vi "PLC.CheckStatus.vi"(7 "Idx":i32, 8 "error in":errorcluster, 10 "Slot":i32, 11 "Data_in":T1={"Status"={"Idx"=0, "ConnRef"=0, "State"=enum."Off", "LiveBitTimer"=timestamp(0 s since 1904-01-01)}, "Sets"={"Enable"=FALSE, "IP"="", "Rack"=0, "Slot"=0, "LifeBitTimer_s"=0.0, "DataBlockAddr_PCStatus"=0, "DataBlockAddr_PLCStatus"=1, "DataBlockAddr_PLCNewData"=[], "DataBlockSize_PLCNewData"=[], "DataBlockAddr_PLCChangeOver"=[], "DataBlockSize_PLCChangeOver"=[], "DataBlockAddr_PCChangeOver"=[], "DataBlockAddr_PLCCheckStatus"=[], "DataBlockSize_PLCCheckStatus"=[], "DataBlockAddr_PCCheckStatus"=[], "System"=""}, "PCstatus"={"General"={"LifeBit"=FALSE, "DbRun"=FALSE}, "Stations"=[]}, "PLCstatus"={"General"={"LifeBit"=FALSE}, "Stations"=[]}}) -> (0 "error out":errorcluster, 3 "Data_out":T1={"Status"={"Idx"=0, "ConnRef"=0, "State"=enum."Off", "LiveBitTimer"=timestamp(0 s since 1904-01-01)}, "Sets"={"Enable"=FALSE, "IP"="", "Rack"=0, "Slot"=0, "LifeBitTimer_s"=0.0, "DataBlockAddr_PCStatus"=0, "DataBlockAddr_PLCStatus"=1, "DataBlockAddr_PLCNewData"=[], "DataBlockSize_PLCNewData"=[], "DataBlockAddr_PLCChangeOver"=[], "DataBlockSize_PLCChangeOver"=[], "DataBlockAddr_PCChangeOver"=[], "DataBlockAddr_PLCCheckStatus"=[], "DataBlockSize_PLCCheckStatus"=[], "DataBlockAddr_PCCheckStatus"=[], "System"=""}, "PCstatus"={"General"={"LifeBit"=FALSE, "DbRun"=FALSE}, "Stations"=[]}, "PLCstatus"={"General"={"LifeBit"=FALSE}, "Stations"=[]}})   [LabVIEW 2016]
doc: "Get test results (measurement values) from PLC and save to database\n\nWabco 2017 All right reserved\nAuthor: maciej.szupienko@wabco-auto.com"
uses:
  PLC.Data.ctl
  PLC.Data.Status.ctl
  PLC.State.ctl
  PLC.Data.Sets.ctl
  LowLevel/PLC.DataBlock.PCstatus.ctl
  LowLevel/PLC.DataBlock.PCstatus.General.ctl
  LowLevel/PLC.DataBlock.PCstatus.Station.ctl
  LowLevel/PLC.DataBlock.PLCstatus.ctl
  LowLevel/PLC.DataBlock.PLCstatus.General.ctl
  LowLevel/PLC.DataBlock.PLCstatus.Station.ctl
  LowLevel/PLC.DataBlock.PLCcheckstatus.ctl
  LowLevel/PLC.DataBlock.PCcheckstatus.ctl
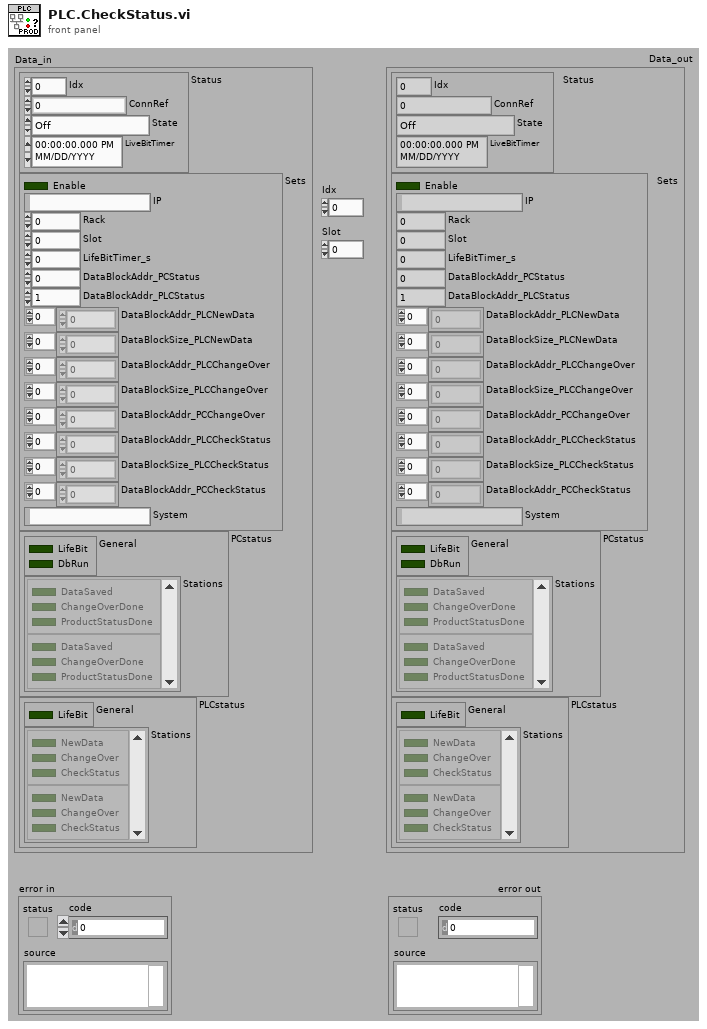
[diagram p1: front panel]
types:
  T1 = typedef "PLC.Data.ctl" = cluster{"Status":T2, "Sets":T4, "PCstatus":T5, "PLCstatus":T8}
  T2 = typedef "PLC.Data.Status.ctl" = cluster{"Idx":i32, "ConnRef":u64, "State":T3, "LiveBitTimer":timestamp}
  T3 = typedef "PLC.State.ctl" = enum32{"Off", "Error", "Idle", "Run"}
  T4 = typedef "PLC.Data.Sets.ctl" = cluster{"Enable":bool, "IP":string, "Rack":i32, "Slot":i32, "LifeBitTimer_s":dbl, "DataBlockAddr_PCStatus":i32, "DataBlockAddr_PLCStatus":i32, "DataBlockAddr_PLCNewData":i32[], "DataBlockSize_PLCNewData":i32[], "DataBlockAddr_PLCChangeOver":i32[], "DataBlockSize_PLCChangeOver":i32[], "DataBlockAddr_PCChangeOver":i32[], "DataBlockAddr_PLCCheckStatus":i32[], "DataBlockSize_PLCCheckStatus":i32[], "DataBlockAddr_PCCheckStatus":i32[], "System":string}
  T5 = typedef "PLC.DataBlock.PCstatus.ctl" = cluster{"General":T6, "Stations":T7[]}
  T6 = typedef "PLC.DataBlock.PCstatus.General.ctl" = cluster{"LifeBit":bool, "DbRun":bool}
  T7 = typedef "PLC.DataBlock.PCstatus.Station.ctl" = cluster{"DataSaved":bool, "ChangeOverDone":bool, "ProductStatusDone":bool}
  T8 = typedef "PLC.DataBlock.PLCstatus.ctl" = cluster{"General":T9, "Stations":T10[]}
  T9 = typedef "PLC.DataBlock.PLCstatus.General.ctl" = cluster{"LifeBit":bool}
  T10 = typedef "PLC.DataBlock.PLCstatus.Station.ctl" = cluster{"NewData":bool, "ChangeOver":bool, "CheckStatus":bool}
  T11 = typedef "PLC.DataBlock.PCcheckstatus.ctl" = cluster{"Ref":string, "Serial":string, "StatusPrev":i8, "StatusThis":i8, "Repetitions":u8}
  T12 = typedef "PLC.DataBlock.PLCcheckstatus.ctl" = cluster{"Ref1":string, "Serial1":string, "Ref2":string, "Serial2":string}
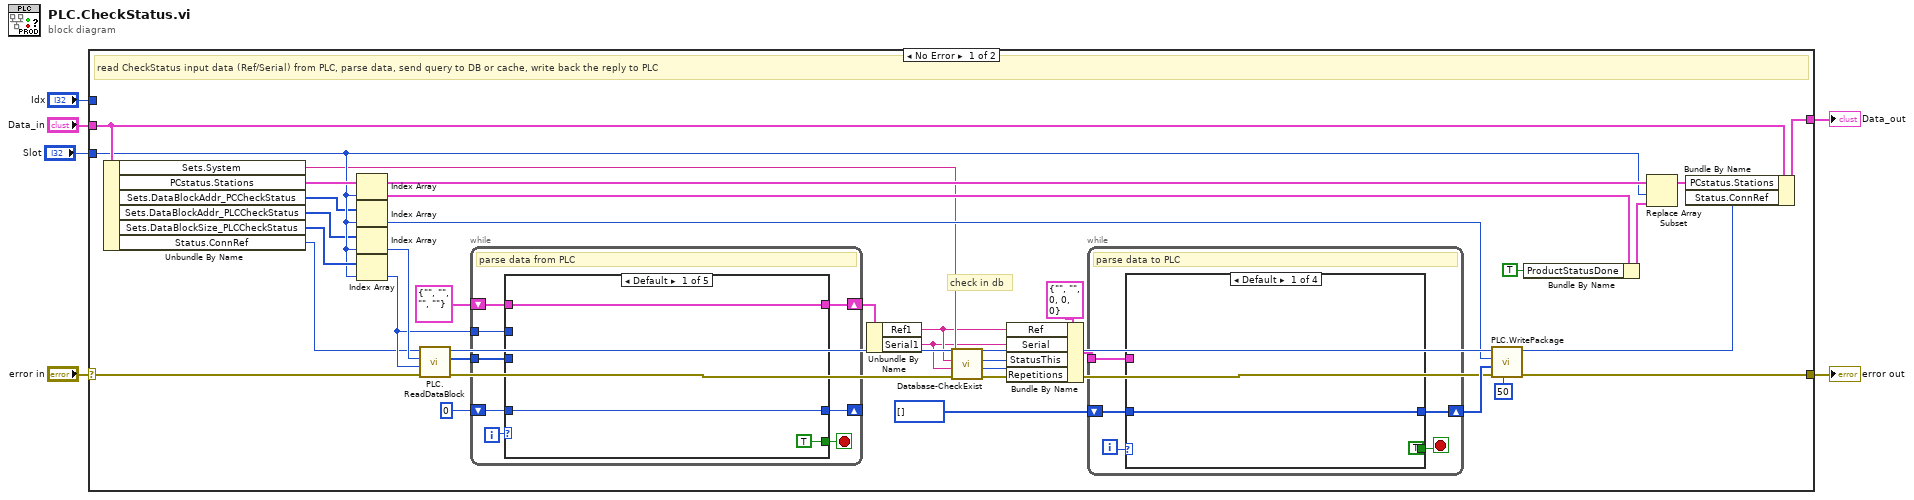
[diagram p0: block diagram]
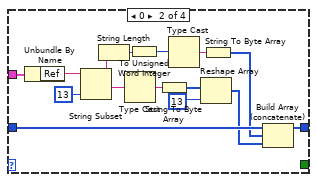
[diagram p2: hidden frame]
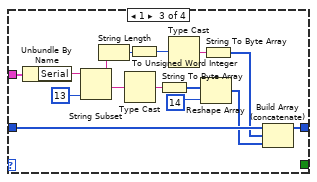
[diagram p3: hidden frame]
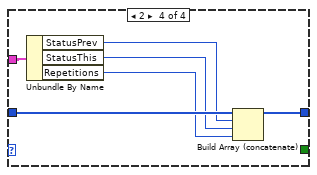
[diagram p4: hidden frame]
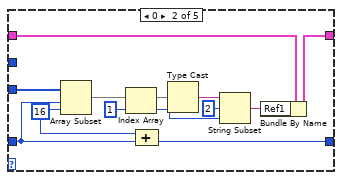
[diagram p5: hidden frame]
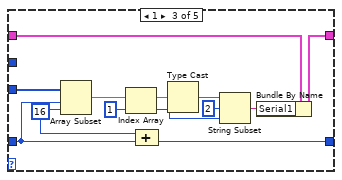
[diagram p6: hidden frame]
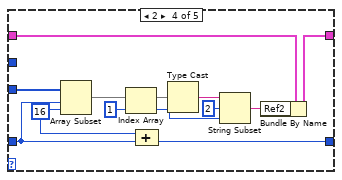
[diagram p7: hidden frame]
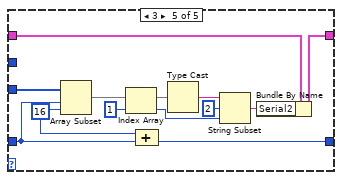
[diagram p8: hidden frame]
diagram:
  n1 = case shown="No Error" "error in" {
    selector: "error in" -> [w40 w143]
    tunnel: [w28 w143] -> w3
    tunnel: "Data_in" -> [w38 w142]
    tunnel: [w41 w142] -> w5
    tunnel: "Idx" -> [_ _]
    tunnel: "Slot" -> [w23 _]
    frame No Error {
      # "check in db"
      # "read CheckStatus input data (Ref/Serial) from PLC, parse data, send query to DB or cache, write back the reply to PLC"
      n2 = Unbundle By Name(w38) -> ("Sets.System"=w15:string, "PCstatus.Stations"=w24:T7[], "Sets.DataBlockAddr_PCCheckStatus"=w19:i32[], "Sets.DataBlockAddr_PLCCheckStatus"=w20:i32[], "Sets.DataBlockSize_PLCCheckStatus"=w30:i32[], "Status.ConnRef"=w18:u64)
      n3 = Index Array(array=w24, index=w23) -> (element=w36:T7)
      n4 = Index Array(array=w19, index=w23) -> (element=w21:i32)
      n5 = Index Array(array=w20, index=w23) -> (element=w39:i32)
      n6 = Index Array(array=w30, index=w23) -> (element=w31:i32)
      n7 = call "PLC.ReadDataBlock.vi"("error in (no error)"=w40, "Amount (1)"=w31, "Block"=w39, "Ref"=w18) -> ("error out"=w14:errorcluster, "data out"=w34:u8[], "ref out"=w29:u64)  [unwired: 5 in]
      n8 = while {
        tunnel: w34 -> [w85]
        shift-right: [w88] -> _
        shift-left: 0 -> [w89]
        shift-right: [w87] -> w16
        shift-left: T12 {"Ref1"="", "Serial1"="", "Ref2"="", "Serial2"=""} ("element") -> [w86]
        tunnel: w31 -> [w84]
        i -> [w90]
        stop <- w83 stop-if-true
        # "parse data from PLC"
        n9 = case shown="Default" w90 {
          tunnel: w89 -> [w92 w96 w108 w120 w132]
          tunnel: [w92 w95 w107 w119 w131] -> w88
          tunnel: [w93 w105 w117 w129 w141] -> w87
          tunnel: w86 -> [w93 w104 w116 w128 w140]
          tunnel: w85 -> [_ w99 w111 w123 w135]
          tunnel: w84 -> [_ _ _ _ _]
          tunnel: [TRUE _ _ _ _] -> w83
          frame Default {
          }
          frame 0 {
            w97 = 16 ("length")
            n10 = Array Subset(array=w99, index=w96, length=w97) -> (w101:u8[])
            n11 = Index Array(array=w101, index=1) -> (element=w94:u8)
            n12 = Compound Arithmetic op=ADD(w97, w96) -> (w95:i32)
            n13 = Type Cast(x=w101) -> (*(type *) &x=w100:string)  [unwired: 1 in]
            n14 = String Subset(string=w100, offset (0)=2, length (rest)=w94) -> (substring=w98:string)
            n15 = Bundle By Name(cluster=w104, "Ref1"=w98) -> (w105:T12)
          }
          frame 1 {
            w109 = 16 ("length")
            n16 = Array Subset(array=w111, index=w108, length=w109) -> (w113:u8[])
            n17 = Index Array(array=w113, index=1) -> (element=w106:u8)
            n18 = Compound Arithmetic op=ADD(w109, w108) -> (w107:i32)
            n19 = Type Cast(x=w113) -> (*(type *) &x=w112:string)  [unwired: 1 in]
            n20 = String Subset(string=w112, offset (0)=2, length (rest)=w106) -> (substring=w110:string)
            n21 = Bundle By Name(cluster=w116, "Serial1"=w110) -> (w117:T12)
          }
          frame 2 {
            w121 = 16 ("length")
            n22 = Array Subset(array=w123, index=w120, length=w121) -> (w125:u8[])
            n23 = Index Array(array=w125, index=1) -> (element=w118:u8)
            n24 = Compound Arithmetic op=ADD(w121, w120) -> (w119:i32)
            n25 = Type Cast(x=w125) -> (*(type *) &x=w124:string)  [unwired: 1 in]
            n26 = String Subset(string=w124, offset (0)=2, length (rest)=w118) -> (substring=w122:string)
            n27 = Bundle By Name(cluster=w128, "Ref2"=w122) -> (w129:T12)
          }
          frame 3 {
            w133 = 16 ("length")
            n28 = Array Subset(array=w135, index=w132, length=w133) -> (w137:u8[])
            n29 = Index Array(array=w137, index=1) -> (element=w130:u8)
            n30 = Compound Arithmetic op=ADD(w133, w132) -> (w131:i32)
            n31 = Type Cast(x=w137) -> (*(type *) &x=w136:string)  [unwired: 1 in]
            n32 = String Subset(string=w136, offset (0)=2, length (rest)=w130) -> (substring=w134:string)
            n33 = Bundle By Name(cluster=w140, "Serial2"=w134) -> (w141:T12)
          }
        }
      }
      n34 = Unbundle By Name(w16) -> ("Ref1"=w11:string, "Serial1"=w7:string)
      n35 = call "Database-CheckExist.vi"("error in"=w14, "Serial"=w7, "Ref"=w11, "System"=w15) -> ("error out"=w13:errorcluster, "Repetitions"=w9:u8, "Status"=w10:i8)  [unwired: 5 in]
      n36 = Bundle By Name(cluster=T11 {"Ref"="", "Serial"="", "StatusPrev"=0, "StatusThis"=0, "Repetitions"=0} ("PCcheckstatus"), "Ref"=w11, "Serial"=w7, "StatusThis"=w10, "Repetitions"=w9) -> (w8:T11)
      n37 = while {
        tunnel: w8 -> [w45]
        shift-right: [w43] -> w26
        shift-left: u8[] [] ("data in") -> [w42]
        i -> [w46]
        stop <- w44 stop-if-true
        # "parse data to PLC"
        n38 = case shown="Default" w46 {
          tunnel: w45 -> [_ w62 w76 w82]
          tunnel: [TRUE _ _ _] -> w44
          tunnel: [w47 w61 w75 w77] -> w43
          tunnel: w42 -> [w47 w60 w74 w81]
          frame Default {
          }
          frame 0 {
            n39 = Unbundle By Name(w62) -> ("Ref"=w58:string)
            n40 = String Subset(string=w58, length (rest)=13 ("length (rest)")) -> (substring=w53:string)  [unwired: 1 in]
            n41 = String Length(string=w53) -> (length=w59:i32)
            n42 = Type Cast(x=w53) -> (*(type *) &x=w54:string)  [unwired: 1 in]
            n43 = To Unsigned Word Integer(number=w59) -> (unsigned 16bit integer=w57:u16)
            n44 = String To Byte Array(string=w54) -> (unsigned byte array=w52:u8[])
            n45 = Type Cast(x=w57) -> (*(type *) &x=w56:string)  [unwired: 1 in]
            n46 = Reshape Array(w52, 13 ("length (rest)")) -> (w51:u8[])
            n47 = String To Byte Array(string=w56) -> (unsigned byte array=w55:u8[])
            n48 = Build Array (concatenate)(w60, w55, w51) -> (w61:u8[])
          }
          frame 1 {
            n49 = Unbundle By Name(w76) -> ("Serial"=w72:string)
            n50 = String Subset(string=w72, length (rest)=13 ("length (rest)")) -> (substring=w67:string)  [unwired: 1 in]
            n51 = String Length(string=w67) -> (length=w73:i32)
            n52 = Type Cast(x=w67) -> (*(type *) &x=w68:string)  [unwired: 1 in]
            n53 = To Unsigned Word Integer(number=w73) -> (unsigned 16bit integer=w71:u16)
            n54 = String To Byte Array(string=w68) -> (unsigned byte array=w66:u8[])
            n55 = Type Cast(x=w71) -> (*(type *) &x=w70:string)  [unwired: 1 in]
            n56 = Reshape Array(w66, 14 ("length (rest)")) -> (w65:u8[])
            n57 = String To Byte Array(string=w70) -> (unsigned byte array=w69:u8[])
            n58 = Build Array (concatenate)(w74, w69, w65) -> (w75:u8[])
          }
          frame 2 {
            n59 = Unbundle By Name(w82) -> ("StatusPrev"=w80:i8, "StatusThis"=w79:i8, "Repetitions"=w78:u8)
            n60 = Build Array (concatenate)(w81, w80, w79, w78) -> (w77:u8[])
          }
        }
      }
      n61 = call "PLC.WritePackage.vi"("max package size  (0: full)"=50, "error in (no error)"=w13, "data"=w26, "addr"=w21, "Ref in"=w29) -> ("error out"=w28:errorcluster, "Ref out"=w25:u64)  [unwired: 5 in]
      n62 = Bundle By Name(cluster=w36, "ProductStatusDone"=TRUE ("ChangeOverDone")) -> (w35:T7)
      n63 = Replace Array Subset(array=w24, new element=w35, index=w23) -> (w37:T7[])
      n64 = Bundle By Name(cluster=w38, "PCstatus.Stations"=w37, "Status.ConnRef"=w25) -> (w41:T1)
    }
    frame Error {
    }
  }
  "error out" <- w3
  "Data_out" <- w5
